vi "边沿计数_位置比较事件导出.vi"() -> ()   [LabVIEW 2013]
doc: "This example demonstrates how to count the pulse's edges."
uses:
  <userlib>/ArtDAQ/_SubVI/ArtDAQ_CreateCICountEdgesChan.vi
  <userlib>/ArtDAQ/_SubVI/ArtDAQ_Read Counter U32 1Samp.vi
panel:
  out "计数值":u32
  in  "输出脉宽(100ns)":u32[](array[numeric])=[1000, 1000, 1000, 1000, 1000, 1000, 1000, 1000, 1000, 1000, 1000, 1000, 1000, 1000, 1000, 1000, 1000, 1000, 1000, 1000, 1000, 1000, 1000, 1000, 1000, 1000, 1000, 1000, 1000, 1000, 1000, 1000, 1000, 1000, 1000, 1000, 1000, 1000, 1000, 1000, 1000, 1000, 1000, 1000, 1000, 1000, 1000, 1000, 1000, 1000, 1000, 1000, 1000, 1000, 1000, 1000, 1000, 1000, 1000, 1000, 1000, 1000, 1000, 1000, 1000, 1000, 1000, 1000, 1000, 1000, 1000, 1000, 1000, 1000, 1000, 1000, 1000, 1000, 1000, 1000, 1000, 1000, 1000, 1000, 1000, 1000, 1000, 1000, 1000, 1000, 1000, 1000, 1000, 1000, 1000, 1000, 1000, 1000, 1000, 1000]
  in  "预设位置数组":u32[](array[numeric])=[0, 1000, 2000, 3000, 4000, 5000, 6000, 7000, 8000, 9000, 10000, 11000, 12000, 13000, 14000, 15000, 16000, 17000, 18000, 19000, 20000, 21000, 22000, 23000, 24000, 25000, 26000, 27000, 28000, 29000, 30000, 31000, 32000, 33000, 34000, 35000, 36000, 37000, 38000, 39000, 40000, 41000, 42000, 43000, 44000, 45000, 46000, 47000, 48000, 49000, 50000, 51000, 52000, 53000, 54000, 55000, 56000, 57000, 58000, 59000, 60000, 61000, 62000, 63000, 64000, 65000, 66000, 67000, 68000, 69000, 70000, 71000, 72000, 73000, 74000, 75000, 76000, 77000, 78000, 79000, 80000, 81000, 82000, 83000, 84000, 85000, 86000, 87000, 88000, 89000, 90000, 91000, 92000, 93000, 94000, 95000, 96000, 97000, 98000, 99000]
  in  "脉宽模式":i32(ring)=10601 items=["隐式"=10601, "预设"=10602]
  in  "输出端口":string="/Dev1/PFI11"
  in  "脉冲输出极性":i32(ring)=10095 items=["高电平"=10095, "低电平"=10096]
  in  "反转空闲状态":i32(ring)=10192 items=["高"=10192, "低"=10214]
  in  "输出方式":i32(ring)=10265 items=["脉冲方式"=10265, "反转方式"=10307]
  in  "计数器":string="Dev1/CTR0"
  in  "停止":bool
  out "错误输出":errorcluster={"status"=FALSE, "code"=0, "source"="\n"}
  # "通道属性"
  # "输出事件"
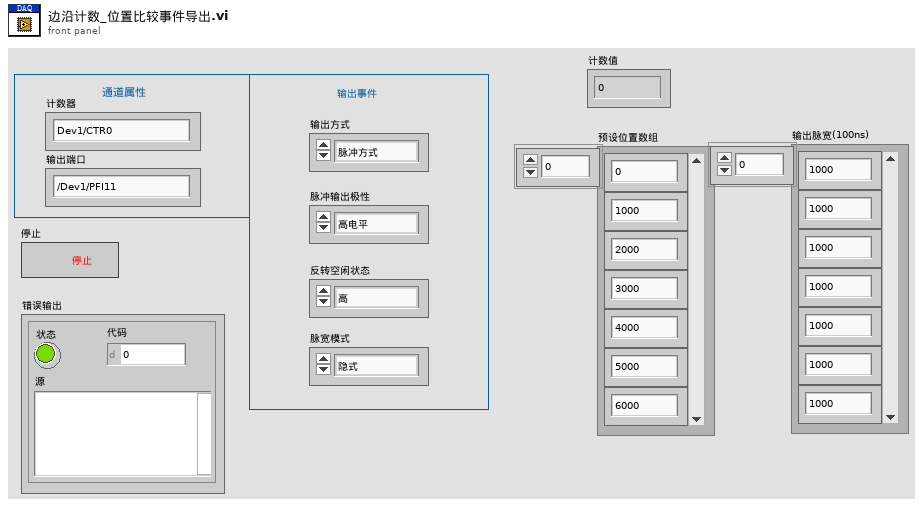
[diagram p1: front panel]
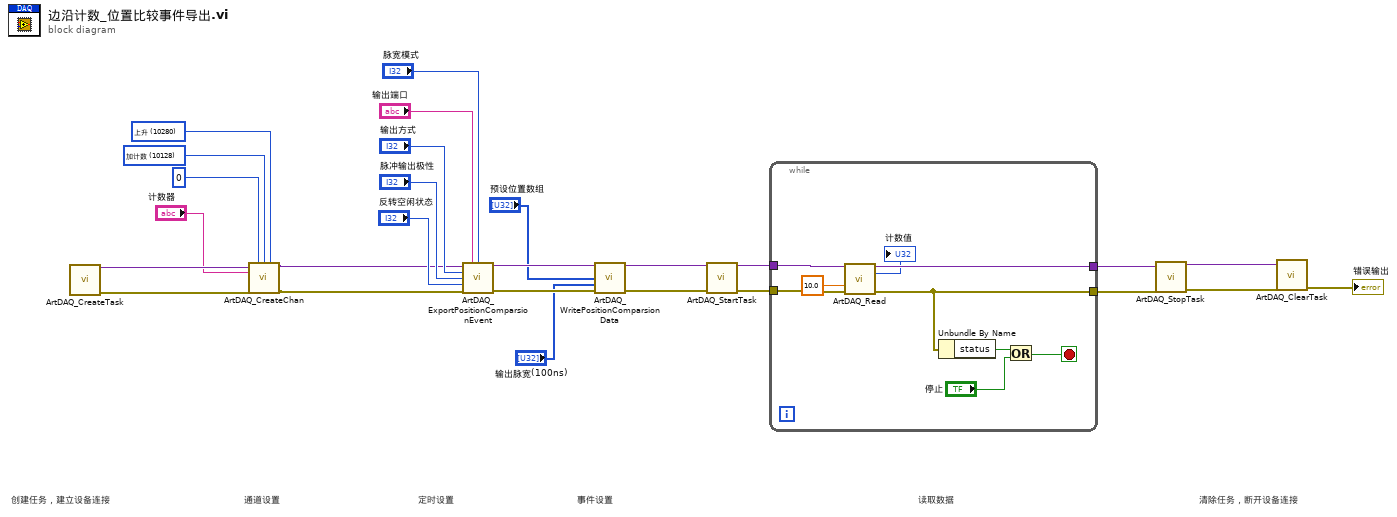
[diagram p0: block diagram]
diagram:
  w22 = 10280 items=["上升"=10280, "下降"=10171] ("计数边沿")
  w23 = 10128 items=["加计数"=10128, "减计数"=10124, "外部控制"=10326] ("计数方式")
  # "清除任务，断开设备连接"
  # "读取数据"
  # "事件设置"
  # "定时设置"
  # "通道设置"
  # "创建任务，建立设备连接"
  n1 = call <userlib>:"ArtDAQ_CreateTask.vi"() -> ("任务句柄"=w26:variant, "错误输出"=w25:errorcluster)  [unwired: 14 in]
  n2 = call-poly <userlib>:"ArtDAQ_CreateChan.vi"("任务句柄"=w26, "初始计数"=u32 0 ("InitialCount"), "计数方向"=w23, "边沿"=w22, "计数器"="计数器", "错误输入"=w25) -> ("任务句柄"=w9:variant, "错误输出"=w8:errorcluster)  [unwired: 8 in]
  n3 = call <userlib>:"ArtDAQ_ExportPositionComparsionEvent.vi"("任务句柄"=w9, "输出接线端"="输出端口", "脉宽模式"="脉宽模式", "输出方式"="输出方式", "脉冲极性"="脉冲输出极性", "反转空闲状态"="反转空闲状态", "ErrorInput"=w8) -> ("任务句柄"=w4:variant, "ErrorOutput"=w6:errorcluster)  [unwired: 7 in]
  n4 = call <userlib>:"ArtDAQ_WritePositionComparsionData.vi"("任务句柄"=w4, "positionArray"="预设位置数组", "pulseWidthArray"="输出脉宽(100ns)", "错误输入"=w6) -> ("任务句柄"=w3:variant, "错误输出"=w5:errorcluster)  [unwired: 9 in, 1 out]
  n5 = call <userlib>:"ArtDAQ_StartTask.vi"("任务句柄"=w3, "错误输入"=w5) -> ("任务句柄"=w15:variant, "错误输出"=w14:errorcluster)  [unwired: 12 in]
  n6 = while {
    tunnel: [w35] -> w20
    tunnel: [w31] -> w18
    tunnel: w15 -> [w34]
    tunnel: w14 -> [w33]
    stop <- w28 stop-if-true
    n7 = call-poly <userlib>:"ArtDAQ_Read.vi"("任务句柄"=w34, "超时s"=10.0 ("Timeout"), "错误输入"=w33) -> ("任务句柄"=w35:variant, "数据"=→"计数值":u32, "错误输出"=w31:errorcluster)  [unwired: 10 in]
    n8 = Unbundle By Name(w31) -> ("status"=w30:bool)
    n9 = Or(x=w30, y="停止") -> (x .or. y?=w28:bool)
  }
  n10 = call <userlib>:"ArtDAQ_StopTask.vi"("任务句柄"=w20, "错误输入"=w18) -> ("任务句柄"=w19:variant, "错误输出"=w17:errorcluster)  [unwired: 12 in]
  n11 = call <userlib>:"ArtDAQ_ClearTask.vi"("任务句柄"=w19, "错误输入"=w17) -> ("错误输出"=→"错误输出":errorcluster)  [unwired: 13 in]
